vi "Modify Point Roi.vi"(11 "ROI in":T1) -> (3 "ROI out":T1)   [LabVIEW 2016]
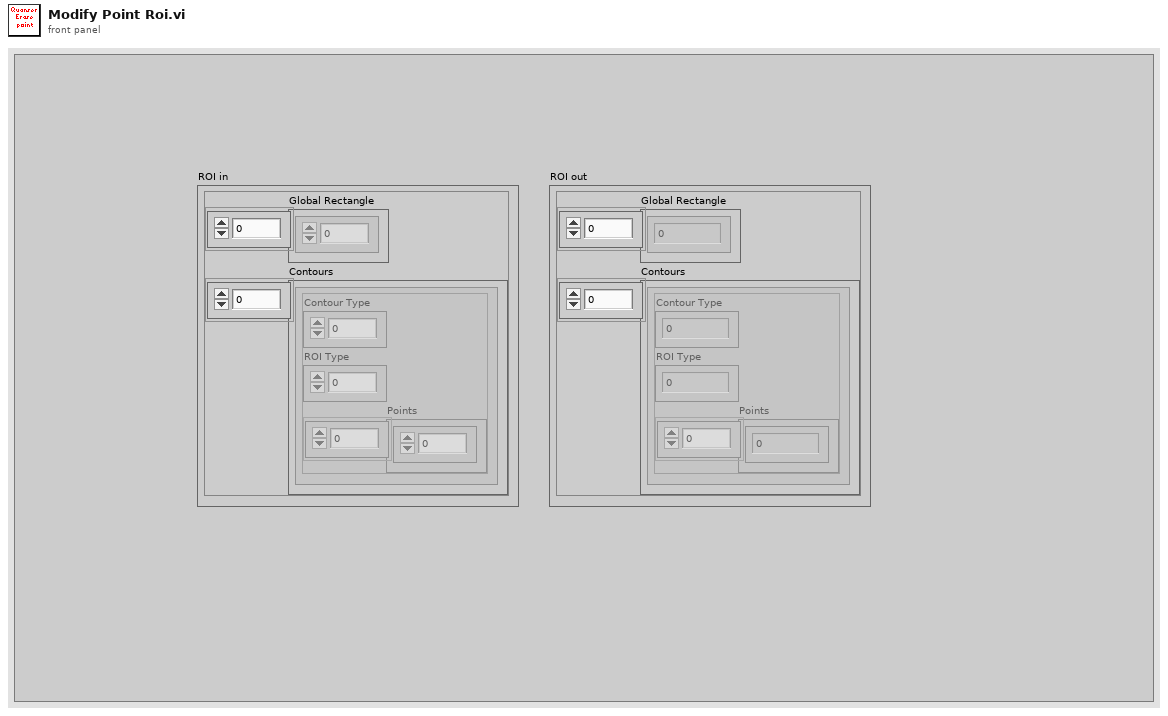
[diagram p1: front panel]
types:
  T1 = cluster{"Global Rectangle":i32[], "Contours":cluster{"Contour Type":u32, "ROI Type":u32, "Points":i32[]}[]}
  T2 = cluster{"Contour Type":u32, "ROI Type":u32, "Points":i32[]}[]
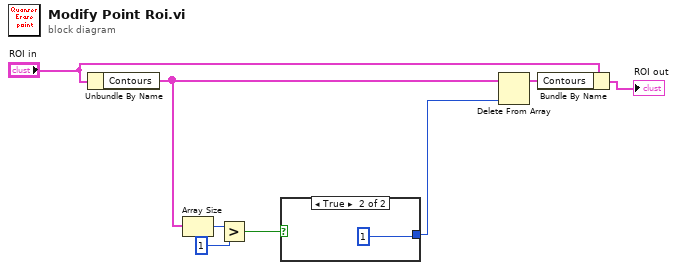
[diagram p0: block diagram]
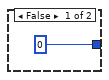
[diagram p2: hidden frame]
diagram:
  n1 = Unbundle By Name("ROI in") -> ("Contours"=w2:T2)
  n2 = Array Size(array=w2) -> (size(s)=w5:i32)
  n3 = Greater?(x=w5, y=1) -> (0:w3:bool)
  n4 = case shown="True" w3 {
    tunnel: [0 ("y") 1 ("y")] -> w1
    frame False {
    }
    frame True {
    }
  }
  n5 = Delete From Array(array=w2, index=w1) -> (array with subset deleted=w6:T2)  [unwired: 1 in, 1 out]
  n6 = Bundle By Name(cluster="ROI in", "Contours"=w6) -> (→"ROI out":T1)
